vi "Results.Evaluate Overall Result Based on Failure Priority.vi"(9 "ConfigDir":path, 11 "Meas":T3[](array[typedef]) {"Status" items=["LOG", "PASS", "FAIL", "ERROR"]}) -> (2 "Change":bool, 3 "ResultState":T1={"State"=enum."Passing", "Code"=0, "Description"=""})   [LabVIEW 2019]
uses:
  Result.Measurement Item.ctl
  Result.Measurement and Attribute Item Status.ctl
  <vilib>/KATE/SeqMgr/SeqMgr.Result Info.ctl
  <vilib>/KATE/SeqMgr/SeqMgr.Result State Enum.ctl
  <vilib>/KATE/SeqMgr/SeqMgr.lvlib
  <vilib>/KATE/Files/File Utils.lvlib
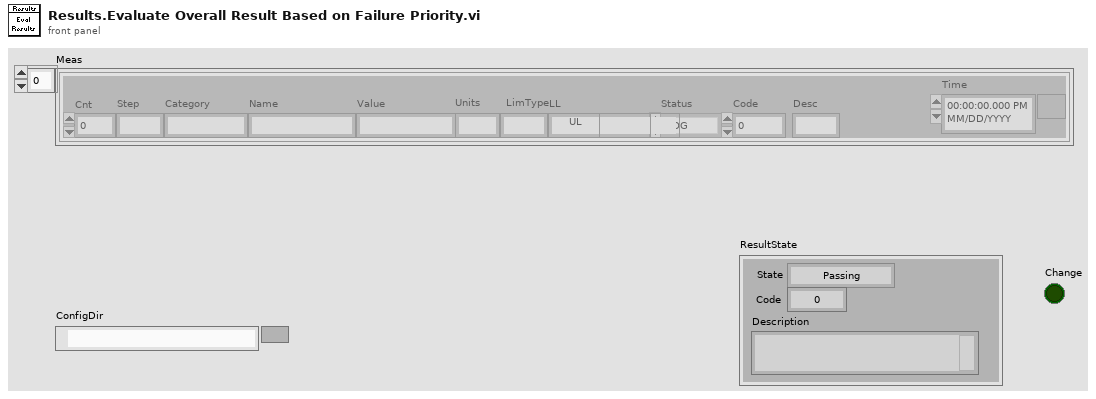
[diagram p1: front panel]
types:
  T1 = typedef "KATE_Lib.lvlib/SeqMgr.lvlib/SeqMgr.Result Info.ctl" = cluster{"State":T2, "Code":i32, "Description":string}
  T2 = typedef "KATE_Lib.lvlib/SeqMgr.lvlib/SeqMgr.Result State Enum.ctl" = enum16{"None", "Passing", "Failing", "PASS", "FAIL", "ABORT", "ERROR"}
  T3 = typedef "Result.Measurement Item.ctl" = cluster{"Cnt":i32, "Step":string, "Category":string, "Name":string, "Value":string, "Units":string, "LimType":string, "LL":string, "UL":string, "Status":T4, "Code":i32, "Desc":string, "Time":timestamp}
  T4 = typedef "Result.Measurement and Attribute Item Status.ctl" = i32
  T5 = cluster{"Names":string[], "Status":T4[], "Codes":i32[], "Descs":string[]}
  T6 = cluster{"Results":cluster{"Names":string[], "Status":T4[], "Codes":i32[], "Descs":string[]}, "Pri":cluster{"Names":string[], "Status":T2[]}, "Changed":bool}
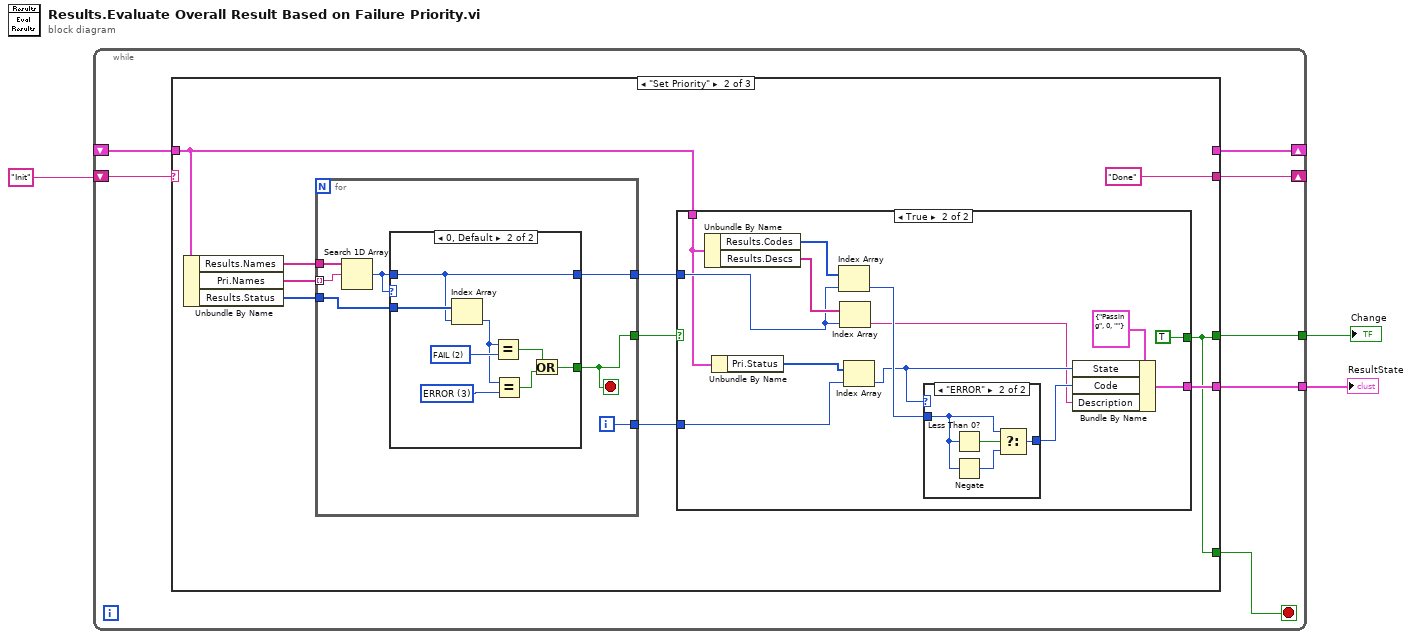
[diagram p0: block diagram]
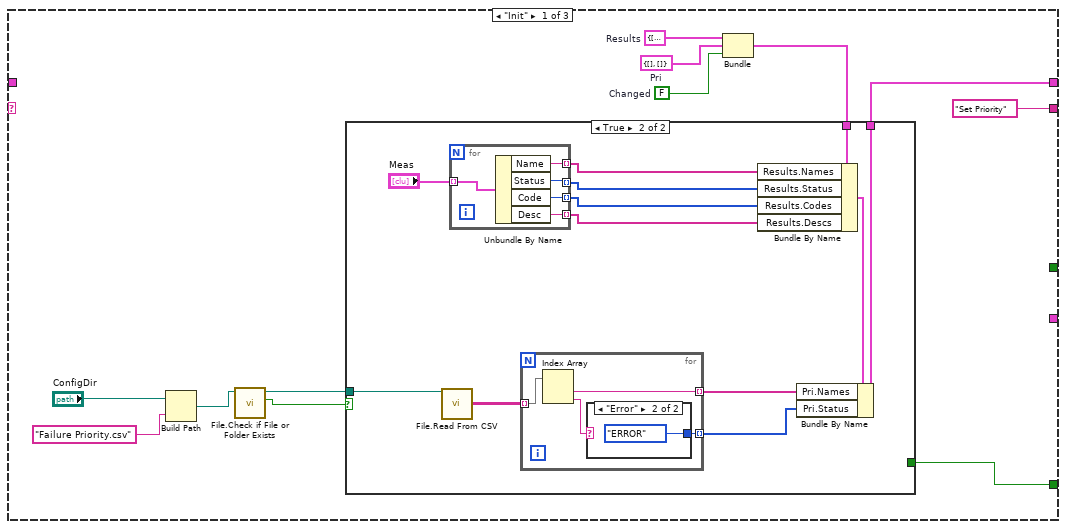
[diagram p2: hidden frame]
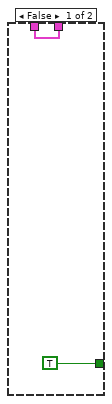
[diagram p3: hidden frame]
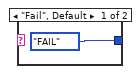
[diagram p4: hidden frame]
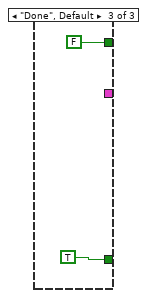
[diagram p8: hidden frame]
diagram:
  n1 = while {
    shift-right: [w9] -> _
    shift-left: "Init" -> [w10]
    tunnel: [w7] -> w2
    tunnel: [w6] -> w1
    shift-right: [w4] -> _
    shift-left: _ -> [w5]
    stop <- w8 stop-if-true
    n2 = case shown="\"Set Priority\"" w10 {
      tunnel: ["Set Priority" "Done" _] -> w9
      tunnel: [w12 w55 TRUE] -> w8
      tunnel: [_ w55 FALSE] -> w7
      tunnel: [_ w56 _] -> w6
      tunnel: w5 -> [_ w50 _]
      tunnel: [w16 _ _] -> w4
      frame "Init" {
        w11 = FALSE  # Changed
        w18 = cluster{"Names":string[], "Status":T2[]} {"Names"=[], "Status"=[]}  # Pri
        w19 = T5 {"Names"=[], "Status"=[], "Codes"=[], "Descs"=[]}  # Results
        n3 = Build Path(base path="ConfigDir", name or relative path="Failure Priority.csv") -> (appended path=w15:path)
        n4 = call <vilib>:"File.Check if File or Folder Exists.vi"("Path"=w15) -> ("Exists"=w13:bool, "Dup Path"=w14:path)  [unwired: 6 in, 3 out]
        n5 = Bundle("Results"=w19, "Pri"=w18, "Changed"=w11) -> (w17:T6)  [unwired: 1 in]
        n6 = case shown="True" w13 {
          tunnel: w17 -> [w24 w32]
          tunnel: [w24 w30] -> w16
          tunnel: w14 -> [_ w25]
          tunnel: [TRUE _] -> w12
          frame False {
          }
          frame True {
            n7 = call <vilib>:"File.Read From CSV.vi"("File"=w25) -> ("Data"=w29:string[][])  [unwired: 8 in, 2 out]
            n8 = for {
              tunnel: "Meas" -> [w47] mode=indexing
              tunnel: [w46] -> w36 mode=indexing
              tunnel: [w45] -> w35 mode=indexing
              tunnel: [w44] -> w34 mode=indexing
              tunnel: [w43] -> w33 mode=indexing
              n9 = Unbundle By Name(w47) -> ("Name"=w46:string, "Status"=w45:T4, "Code"=w44:i32, "Desc"=w43:string)
            }
            n10 = for {
              tunnel: w29 -> [w40] mode=indexing
              tunnel: [w39] -> w28 mode=indexing
              tunnel: [w37] -> w27 mode=indexing
              n11 = Index Array(array=w40) -> (element #1=w39:string, element #2=w38:string)  [unwired: 2 in]
              n12 = case shown="\"Error\"" w38 {
                tunnel: [SeqMgr.Result_State_Enum."FAIL" ("State") SeqMgr.Result_State_Enum."ERROR" ("State")] -> w37
                frame "Fail", Default {
                }
                frame "Error" {
                }
              }
            }
            n13 = Bundle By Name(cluster=w32, "Results.Names"=w36, "Results.Status"=w35, "Results.Codes"=w34, "Results.Descs"=w33) -> (w31:T6)
            n14 = Bundle By Name(cluster=w31, "Pri.Names"=w28, "Pri.Status"=w27) -> (w30:T6)
          }
        }
      }
      frame "Set Priority" {
        n15 = Unbundle By Name(w50) -> ("Results.Names"=w53:string[], "Pri.Names"=w52:string[], "Results.Status"=w51:T4[])
        n16 = for {
          tunnel: [w60] -> w54
          tunnel: w53 -> [w64]
          tunnel: w52 -> [w63] mode=indexing
          tunnel: w51 -> [w62]
          tunnel: [w59] -> w49
          tunnel: [w58] -> w48
          i -> [w58]
          stop <- w60 stop-if-true
          n17 = Search 1D Array(1D array=w64, element=w63) -> (index of element=w61:i32)  [unwired: 1 in]
          n18 = case shown="0, Default" w61 {
            tunnel: w61 -> [_ w65]
            tunnel: w62 -> [_ w71]
            tunnel: [_ w66] -> w60
            tunnel: [_ w65] -> w59
            frame -1 {
            }
            frame 0, Default {
              w69 = T4 3 items=["LOG", "PASS", "FAIL", "ERROR"] ("y")
              w72 = T4 2 items=["LOG", "PASS", "FAIL", "ERROR"] ("y")
              n19 = Index Array(array=w71, index=w65) -> (element=w70:T4)
              n20 = Equal?(x=w70, y=w72) -> (x = y?=w68:bool)
              n21 = Equal?(x=w70, y=w69) -> (x = y?=w67:bool)
              n22 = Or(x=w68, y=w67) -> (x .or. y?=w66:bool)
            }
          }
        }
        n23 = case shown="True" w54 {
          tunnel: [_ w84] -> w56
          tunnel: [_ TRUE] -> w55
          tunnel: w50 -> [_ w78]
          tunnel: w49 -> [_ w79]
          tunnel: w48 -> [_ w76]
          frame False {
          }
          frame True {
            n24 = Unbundle By Name(w78) -> ("Results.Codes"=w81:i32[], "Results.Descs"=w80:string[])
            n25 = Unbundle By Name(w78) -> ("Pri.Status"=w77:T2[])
            n26 = Index Array(array=w81, index=w79) -> (element=w75:i32)
            n27 = Index Array(array=w80, index=w79) -> (element=w73:string)
            n28 = Index Array(array=w77, index=w76) -> (element=w74:T2)
            n29 = case shown="\"ERROR\"" w74 {
              tunnel: [w86 w88] -> w82
              tunnel: w75 -> [w86 w87]
              frame Default {
              }
              frame "ERROR" {
                n30 = Less Than 0?(x=w87) -> (x < 0?=w90:bool)
                n31 = Negate(x=w87) -> (-x=w89:i32)
                n32 = Select(t=w87, s=w90, f=w89) -> (s? t:f=w88:i32)
              }
            }
            n33 = Bundle By Name(cluster=T1 {"State"=enum."Passing", "Code"=0, "Description"=""} ("ResultState"), "State"=w74, "Code"=w82, "Description"=w73) -> (w84:T1)
          }
        }
      }
      frame "Done", Default {
      }
    }
  }
  "ResultState" <- w1
  "Change" <- w2
